vi "GetLines.vi"(8 "error in (no error)":errorcluster, 11 "reference in":refnum<class "Console.lvclass">) -> (0 "error out":errorcluster, 2 "Lines":string, 3 "reference out":refnum<class "Console.lvclass">)   [LabVIEW 2018, in "Console.lvclass"]
doc: "Get all the lines currently on the console"
uses:
  Console.lvclass
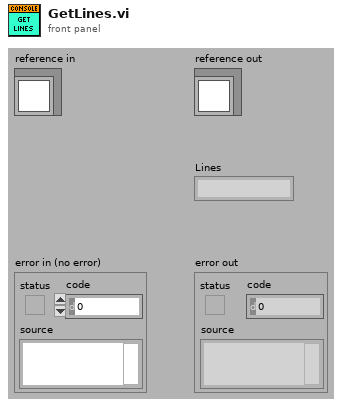
[diagram p1: front panel]
types:
  T1 = typedef "Console.lvclass/ObjectAttributes.ctl" = cluster{"data":string, "count":dbl}
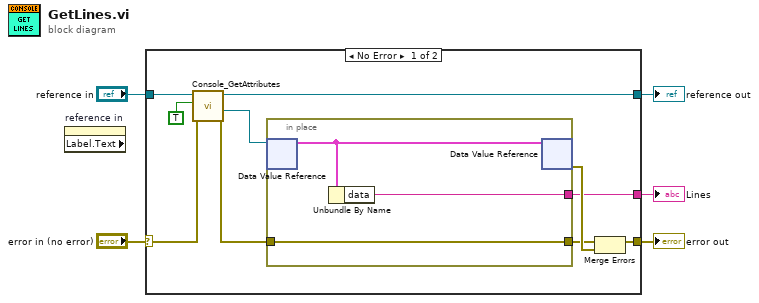
[diagram p0: block diagram]
diagram:
  n1 = property on="reference in" class="LVClassControl (strict)" props=["Label", "Text"]() -> ()  [unwired: 2 in, 3 out]
  n2 = case shown="No Error" "error in (no error)" {
    selector: "error in (no error)" -> [w10 w20]
    tunnel: [w14 w20] -> w4
    tunnel: [w12 w19] -> w2
    tunnel: "reference in" -> [w13 w19]
    tunnel: [w6 _] -> w1
    frame No Error {
      n3 = call "Console_GetAttributes.vi"("error in (no error)"=w10, "OnlyGetDvrReference(False)"=TRUE, "reference in"=w13) -> ("error out"=w9:errorcluster, "DataRef"=w11:refnum<data-value>, "reference out"=w12:refnum<class "Console.lvclass">)  [unwired: 5 in, 1 out]
      n4 = in-place {
        in-place-border: w9 -> [w18]
        in-place-border: [w18] -> w8
        in-place-border: [w16] -> w6
        n5 = in-place-dvr #1(w11) -> (w17:T1)  [unwired: 1 out]
        n6 = Unbundle By Name(w17) -> ("data"=w16:string)
        n7 = in-place-dvr #1(w17) -> (w15:errorcluster)  [unwired: 1 out]
      }
      n8 = Merge Errors(w8, w15) -> (w14:errorcluster)
    }
    frame Error {
    }
  }
  "error out" <- w4
  "reference out" <- w2
  "Lines" <- w1
